vi "Init.vi"(8 "error in (no error)":errorcluster) -> (0 "error out":errorcluster)   [LabVIEW 2017]
uses:
  Controls/Console Select.ctl
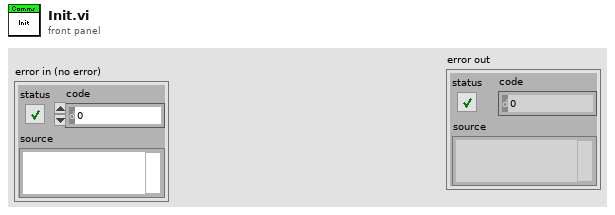
[diagram p1: front panel]
types:
  T1 = typedef "Console Select.ctl" = enum16{"P31 EFX800", "AMT"}
  T2 = enum16{"Init", "Get Index", "Analyze Part", "Analyze Prts", "Analyze Prta", "Set VER", "Set TYPE"}
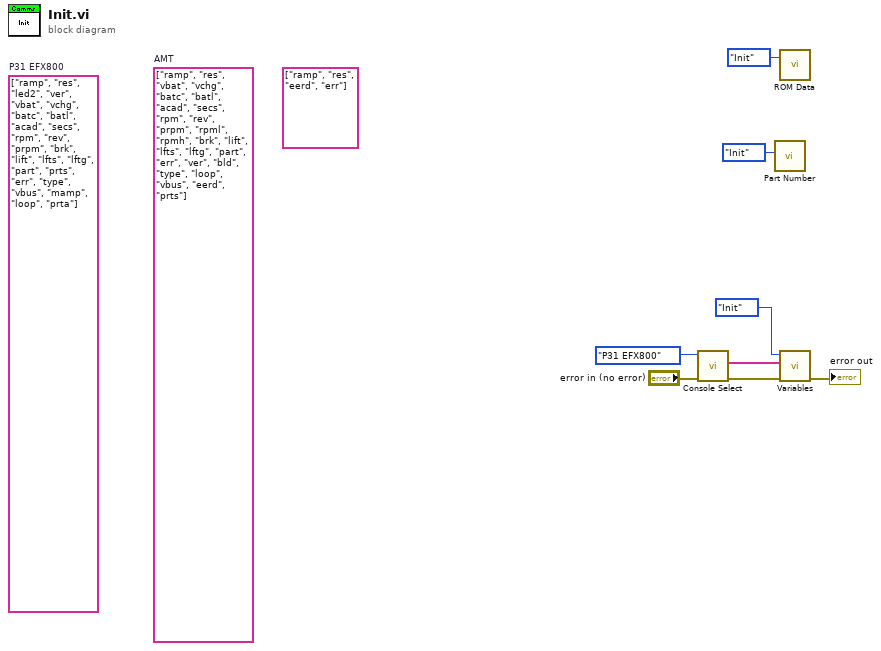
[diagram p0: block diagram]
diagram:
  (unwired) string[] ["ramp", "res", "led2", "ver", "vbat", "vchg", "batc", "batl", "acad", "secs", "rpm", "rev", "prpm", "brk", "lift", "lfts", "lftg", "part", "prts", "err", "type", "vbus", "mamp", "loop", "prta"]  # P31 EFX800
  (unwired) string[] ["ramp", "res", "eerd", "err"]
  (unwired) string[] ["ramp", "res", "vbat", "vchg", "batc", "batl", "acad", "secs", "rpm", "rev", "prpm", "rpml", "rpmh", "brk", "lift", "lfts", "lftg", "part", "err", "ver", "bld", "type", "loop", "vbus", "eerd", "prts"]  # AMT
  n1 = call "Console Select.vi"("error in (no error)"="error in (no error)", "Console Select"=Console_Select."P31 EFX800") -> ("error out"=w4:errorcluster, "Console Out"=w1:string[])  [unwired: 7 in]
  n2 = call "Part Number.vi"("Command"=T2."Init") -> ()  [unwired: 5 in, 6 out]
  n3 = call "ROM Data.vi"("Command"=enum16{"Init", "Get Index", "Analyze"}."Init") -> ()  [unwired: 1 in, 2 out]
  n4 = call "Variables.vi"("error in (no error)"=w4, "Value"=w1, "Command"=enum16{"Init", "Get", "Set Step Counter"}."Init") -> ("error out"=→"error out":errorcluster)  [unwired: 6 in, 2 out]
